vi "CameraControler Analyze.vi"(9 "Climbing Manual Enabled":bool, 11 "JoystickDevRef":T1) -> (0 "Throttle":dbl, 1 "axis 3 (rotation)":dbl, 2 "Y":dbl, 4 "stop auto camera movement":bool, 5 "Center on Target":bool, 7 "View Ground":bool)   [LabVIEW 2012]
uses:
  <vilib>/Rock Robotics/WPI/Joystick/WPI_JoystickDevRef.ctl
  <vilib>/Rock Robotics/WPI/Joystick/WPI_JoystickDeviceEnum.ctl
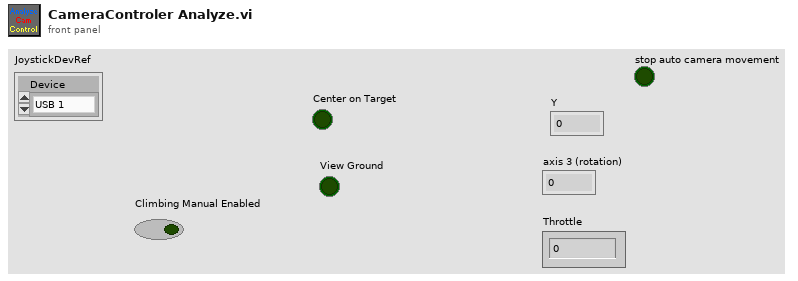
[diagram p1: front panel]
types:
  T1 = typedef "WPI_JoystickDevRef.ctl" = cluster{"Device":T2}
  T2 = typedef "WPI_JoystickDeviceEnum.ctl" = enum16{"USB 1", "USB 2", "USB 3", "USB 4", "Kinect 1", "Kinect 2"}
  T3 = typedef "WPI_JoystickButtonState.ctl" = cluster{"Button 1":bool, "Button 2":bool, "Button 3":bool, "Button 4":bool, "Button 5":bool, "Button 6":bool, "Button 7":bool, "Button 8":bool, "Button 9":bool, "Button 10":bool, "Button 11":bool, "Button 12":bool}
  T4 = cluster{"axis 1 (x)":dbl, "axis 2 (y)":dbl, "axis 3 (throttle)":dbl, "axis 4":dbl, "axis 5":dbl, "axis 6":dbl}
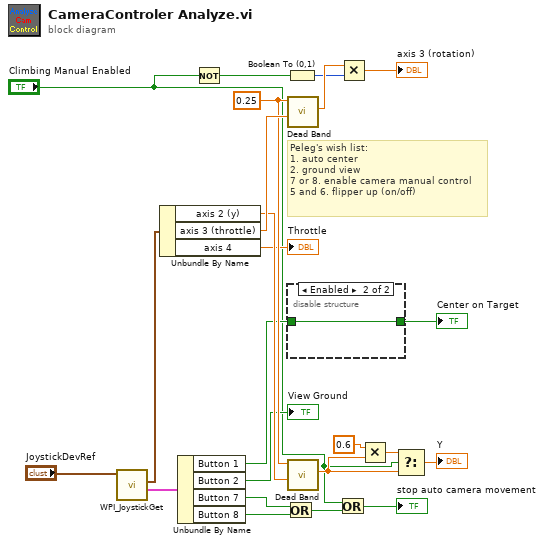
[diagram p0: block diagram]
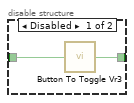
[diagram p2: hidden frame]
diagram:
  w19 = 0.25 ("Dead Band")
  # "Peleg's wish list:\n1. auto center\n2. ground view\n7 or 8. enable camera manual control\n5 and 6. flipper up (on/off)"
  n1 = call <vilib>:"WPI_JoystickGet.vi"("JoystickDevRef"="JoystickDevRef") -> ("Buttons"=w21:T3, "Axes"=w22:T4)  [unwired: 4 in, 1 out]
  n2 = Unbundle By Name(w22) -> ("axis 2 (y)"=w18:dbl, "axis 3 (throttle)"=w20:dbl, "axis 4"=→"Throttle":dbl)
  n3 = Unbundle By Name(w21) -> ("Button 1"=w14:bool, "Button 2"=→"View Ground":bool, "Button 7"=w4:bool, "Button 8"=w3:bool)
  n4 = Not(x="Climbing Manual Enabled") -> (.not. x?=w12:bool)
  n5 = Or(x=w4, y=w3) -> (x .or. y?=w2:bool)
  n6 = Boolean To (0,1)(Boolean=w12) -> (0, 1=w10:i16)
  n7 = call "Dead Band.vi"("Axis In"=w20, "Dead Band"=w19) -> ("Axis Out"=w16:dbl)  [unwired: 9 in]
  n8 = disable-structure shown="Enabled" {
    disable-tunnel: [w25 w26] -> w15
    disable-tunnel: w14 -> [w24 w26]
    frame Disabled {
      n9 = call "Button To Toggle Vr3.vi"("InValue"=w24) -> ("Result"=w25:bool)
    }
    frame Enabled {
    }
  }
  "Center on Target" <- w15
  n10 = call "Dead Band.vi"("Axis In"=w18, "Dead Band"=w19) -> ("Axis Out"=w7:dbl)  [unwired: 9 in]
  n11 = Or(x="Climbing Manual Enabled", y=w2) -> (x .or. y?=→"stop auto camera movement":bool)
  n12 = Multiply(x=w16, y=w10) -> (x*y=→"axis 3 (rotation)":dbl)
  n13 = Multiply(x=0.6, y=w7) -> (x*y=w6:dbl)
  n14 = Select(t=w6, s="Climbing Manual Enabled", f=w7) -> (s? t:f=→"Y":dbl)
